vi "WriteFeedForward.vi"(8 "Memory block":T1, 9 "values Q":dbl[](array[numeric]), 10 "values I":dbl[](array[numeric]), 11 "FPGA VI Reference":T2) -> (3 "FPGA VI Reference Out":T2)   [LabVIEW 2013]
uses:
  Config/FPGAref_5782_FeedForward.ctl
  controls/Memory block.ctl
  <vilib>/rvi/interface/common/niFpgaWaitOnOcc.vi
  <vilib>/Utility/error.llb/Error Cluster From Error Code.vi
  <vilib>/rvi/errors/niLvFpgaAdjustHostInterfaceError.vi
  <vilib>/rvi/interface/nirviMethod/nirviMethod.xnode
  <userlib>/_OpenG.lib/numeric/numeric.llb/Random Number Within Range - DBL__ogtk.vi
  <vilib>/FPGAPlugInAG/Dynamic/niLvFpga_WriteFifo_Dynamic.vi
  <vilib>/rvi/errors/niLvFpgaMergeErrorWithErrorCode.vi
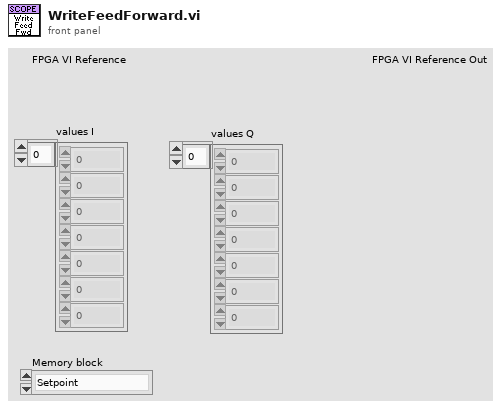
[diagram p1: front panel]
types:
  T1 = typedef "Memory block.ctl" = enum16{"Setpoint", "Beam"}
  T2 = typedef "FPGAref_5782_FeedForward.ctl" = refnum<k20>
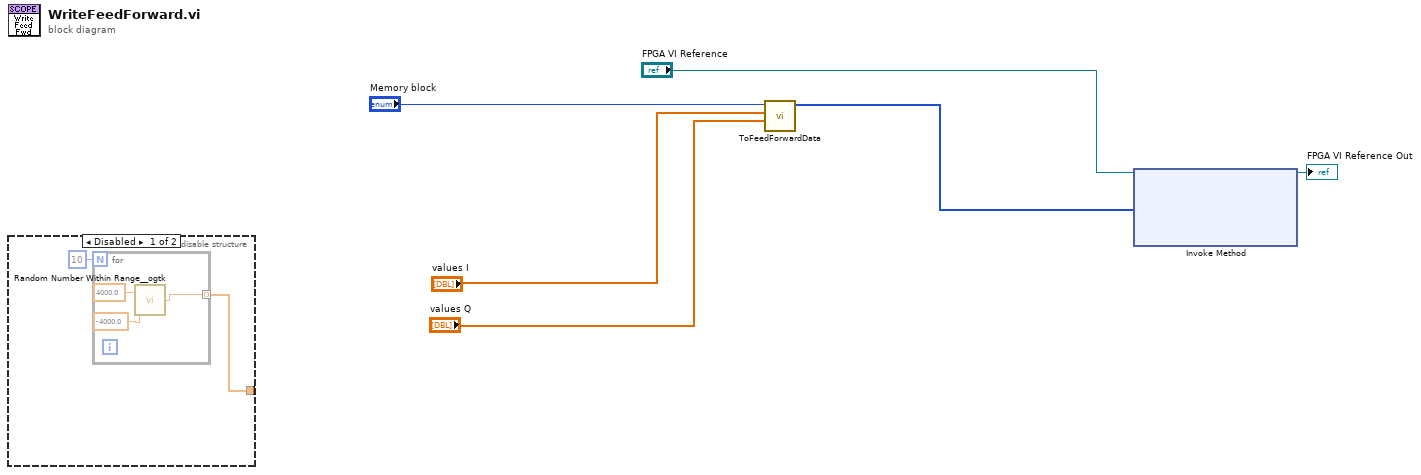
[diagram p0: block diagram]
diagram:
  n1 = disable-structure shown="Disabled" {
    disable-tunnel: [w7 _] -> _
    frame Disabled {
      n2 = for {
        N: 10 -> [_]
        tunnel: [w9] -> w7 mode=indexing
        n3 = call-poly <userlib>:"Random Number Within Range__ogtk.vi"("High"=4000.0, "Low"=-4000.0 ("High")) -> ("Random Number"=w9:dbl)  [unwired: 3 in]
      }
    }
    frame Enabled {
    }
  }
  n4 = call "ToFeedForwardData.vi"("values Q"="values Q", "values I"="values I", "Memory block"="Memory block") -> ("Data"=w3:u64[])  [unwired: 8 in]
  n5 = xnode "Invoke Method"("FPGA VI Reference In"="FPGA VI Reference", "Data"=w3) -> ("FPGA VI Reference Out"=→"FPGA VI Reference Out":T2)  [unwired: 2 in, 2 out]
